vi "OverlayFGENFunctions.vi"() -> ()   [LabVIEW 2023]
doc: "This example shows how to use the Arbitrary Waveform mode to generate on two channels."
uses:
  <instrlib>/niFgen/niFgen.llb/niFgen Output Mode.ctl
  <instrlib>/niFgen/niFgen.llb/niFgen Write Waveform.vi
panel:
  in  "CH0 Waveform Information":cluster{"Waveform Type":u16, "Amplitude":dbl}={"Waveform Type"=0, "Amplitude"=1.0} {"Amplitude" min=0.0 max=1.0 format="%.2f"; "Waveform Type" items=["Sine", "Cosine", "Triangle", "Square", "Sawtooth", "Increasing Ramp", "Decreasing Ramp", "DC Value"]}
  in  "# of points":u32=256
  in  "Update":bool
  in  "Stop":bool
  in  "CH1 Gain":dbl(knob)=0.5 min=0.0 max=2.5 scale=0.0..2.5 scale format="%#.1f"
  in  "CH0 Gain":dbl(knob)=0.5 min=0.0 max=2.5 scale=0.0..2.5 scale format="%#.1f"
  in  "CH1 Waveform Information":cluster{"Waveform Type":u16, "Amplitude":dbl}={"Waveform Type"=1, "Amplitude"=1.0} {"Amplitude" min=0.0 max=1.0 format="%.2f"; "Waveform Type" items=["Sine", "Cosine", "Triangle", "Square", "Sawtooth", "Increasing Ramp", "Decreasing Ramp", "DC Value"]}
  in  "Sample Rate (S/s)":dbl=20000000.0 format="%.2p"
  in  "Sample Clock Source":string(combo)="OnboardClock"
  in  "FGEN Resource Name":refnum<k15>
  out "Waveforms":dbl[][](graph)=[[0.0, 0.024541228522912288, 0.049067674327418015, 0.07356456359966743, 0.0980171403295606, 0.1224106751992162, 0.14673047445536175, 0.17096188876030122, 0.19509032201612828, 0.2191012401568698, 0.2429801799032639, 0.26671275747489837, 0.2902846772544624, 0.31368174039889146, 0.33688985339222005, 0.3598950365349881, 0.3826834323650898, 0.40524131400498986, 0.4275550934302821, 0.4496113296546066, 0.47139673682599764, 0.49289819222978404, 0.5141027441932218, 0.5349976198870973, 0.5555702330196023, 0.5758081914178453, 0.5956993044924334, 0.6152315905806269, 0.6343932841636455, 0.6531728429537769, 0.6715589548470184, 0.689540544737067, 0.7071067811865476, 0.724247082951467, 0.7409511253549591, 0.7572088465064847, 0.773010453362737, 0.7883464276266063, 0.8032075314806449, 0.8175848131515838, 0.8314696123025452, 0.8448535652497072, 0.8577286100002721, 0.8700869911087116, 0.881921264348355, 0.8932243011955154, 0.9039892931234433, 0.9142097557035308, 0.9238795325112867, 0.9329927988347391, 0.9415440651830208, 0.9495281805930369, 0.9569403357322089, 0.9637760657954401, 0.9700312531945441, 0.9757021300385287, 0.9807852804032305, 0.9852776423889413, 0.989176509964781, 0.9924795345987101, 0.9951847266721969, 0.9972904566786903, 0.9987954562051724, 0.9996988186962044, 1.0, 0.9996988186962044, 0.9987954562051724, 0.9972904566786903, 0.9951847266721969, 0.9924795345987101, 0.989176509964781, 0.9852776423889413, 0.9807852804032305, 0.9757021300385286, 0.9700312531945441, 0.9637760657954398, 0.9569403357322089, 0.9495281805930367, 0.9415440651830208, 0.9329927988347388, 0.9238795325112867, 0.9142097557035306, 0.9039892931234433, 0.8932243011955152, 0.881921264348355, 0.8700869911087113, 0.8577286100002721, 0.844853565249707, 0.8314696123025452, 0.8175848131515836, 0.8032075314806449, 0.7883464276266061, 0.773010453362737, 0.7572088465064843, 0.7409511253549591, 0.7242470829514667, 0.7071067811865476, 0.6895405447370667, 0.6715589548470184, 0.6531728429537765, 0.6343932841636455, 0.6152315905806266, 0.5956993044924334, 0.575808191417845, 0.5555702330196023, 0.5349976198870969, 0.5141027441932218, 0.49289819222978376, 0.4713967368259977, 0.4496113296546063, 0.42755509343028214, 0.4052413140049896, 0.38268343236508984, 0.3598950365349879, 0.3368898533922201, 0.31368174039889124, 0.29028467725446244, 0.26671275747489814, 0.24298017990326395, 0.21910124015686955, 0.19509032201612833, 0.17096188876030097, 0.1467304744553618, 0.12241067519921595, 0.09801714032956065, 0.07356456359966718, 0.04906767432741806, 0.024541228522912045, 3.836381624704177e-17, -0.024541228522912528, -0.04906767432741798, -0.07356456359966766, -0.09801714032956058, -0.12241067519921643, -0.14673047445536172, -0.17096188876030144, -0.19509032201612825, -0.21910124015687, -0.24298017990326387, -0.2667127574748986, -0.29028467725446233, -0.3136817403988917, -0.33688985339222, -0.35989503653498833, -0.3826834323650897, -0.40524131400499, -0.42755509343028203, -0.44961132965460676, -0.4713967368259976, -0.4928981922297842, -0.5141027441932217, -0.5349976198870974, -0.5555702330196022, -0.5758081914178454, -0.5956993044924334, -0.6152315905806269, -0.6343932841636455, -0.6531728429537769, -0.6715589548470184, -0.689540544737067, -0.7071067811865476, -0.724247082951467, -0.7409511253549591, -0.7572088465064846, -0.773010453362737, -0.7883464276266062, -0.8032075314806449, -0.8175848131515836, -0.8314696123025452, -0.844853565249707, -0.8577286100002721, -0.8700869911087113, -0.881921264348355, -0.8932243011955152, -0.9039892931234433, -0.9142097557035306, -0.9238795325112867, -0.9329927988347388, -0.9415440651830208, -0.9495281805930366, -0.9569403357322089, -0.9637760657954397, -0.9700312531945441, -0.9757021300385283, -0.9807852804032305, -0.985277642388941, -0.989176509964781, -0.9924795345987097, -0.9951847266721969, -0.99729045667869, -0.9987954562051724, -0.999698818696204, -1.0, -0.999698818696204, -0.9987954562051724, -0.99729045667869, -0.9951847266721969, -0.9924795345987097, -0.989176509964781, -0.985277642388941, -0.9807852804032305, -0.9757021300385283, -0.9700312531945441, -0.9637760657954396, -0.9569403357322089, -0.9495281805930365, -0.9415440651830208, -0.9329927988347386, -0.9238795325112867, -0.9142097557035304, -0.9039892931234433, -0.893224301195515, -0.881921264348355, -0.8700869911087111, -0.8577286100002721, -0.8448535652497068, -0.8314696123025452, -0.8175848131515834, -0.8032075314806449, -0.7883464276266059, -0.773010453362737, -0.7572088465064842, -0.7409511253549591, -0.7242470829514666, -0.7071067811865476, -0.6895405447370666, -0.6715589548470184, -0.6531728429537764, -0.6343932841636455, -0.6152315905806265, -0.5956993044924334, -0.5758081914178449, -0.5555702330196023, -0.5349976198870968, -0.5141027441932218, -0.49289819222978365, -0.4713967368259977, -0.4496113296546062, -0.42755509343028214, -0.4052413140049895, -0.38268343236508984, -0.3598950365349878, -0.3368898533922201, -0.31368174039889113, -0.29028467725446244, -0.26671275747489803, -0.24298017990326395, -0.21910124015686946, -0.19509032201612833, -0.1709618887603009, -0.1467304744553618, -0.1224106751992159, -0.09801714032956066, -0.07356456359966715, -0.04906767432741807, -0.024541228522912028], [1.0, 0.9996988186962042, 0.9987954562051724, 0.9972904566786902, 0.9951847266721969, 0.99247953459871, 0.989176509964781, 0.9852776423889412, 0.9807852804032305, 0.9757021300385286, 0.9700312531945441, 0.9637760657954398, 0.9569403357322089, 0.9495281805930367, 0.9415440651830208, 0.9329927988347388, 0.9238795325112867, 0.9142097557035306, 0.9039892931234433, 0.8932243011955152, 0.881921264348355, 0.8700869911087113, 0.8577286100002721, 0.844853565249707, 0.8314696123025453, 0.8175848131515836, 0.803207531480645, 0.7883464276266061, 0.7730104533627371, 0.7572088465064845, 0.7409511253549592, 0.7242470829514668, 0.7071067811865477, 0.6895405447370668, 0.6715589548470186, 0.6531728429537766, 0.6343932841636456, 0.6152315905806267, 0.5956993044924335, 0.5758081914178451, 0.5555702330196024, 0.534997619887097, 0.5141027441932219, 0.49289819222978387, 0.4713967368259978, 0.44961132965460643, 0.42755509343028225, 0.4052413140049897, 0.38268343236508995, 0.359895036534988, 0.3368898533922202, 0.31368174039889135, 0.29028467725446255, 0.26671275747489825, 0.24298017990326407, 0.2191012401568697, 0.19509032201612844, 0.17096188876030113, 0.14673047445536191, 0.12241067519921611, 0.09801714032956077, 0.07356456359966734, 0.04906767432741818, 0.02454122852291222, 1.655136260252793e-16, -0.024541228522912347, -0.04906767432741785, -0.07356456359966747, -0.09801714032956044, -0.12241067519921624, -0.14673047445536158, -0.17096188876030124, -0.1950903220161281, -0.2191012401568698, -0.24298017990326373, -0.26671275747489837, -0.2902846772544622, -0.31368174039889146, -0.3368898533922199, -0.3598950365349881, -0.3826834323650896, -0.4052413140049898, -0.4275550934302819, -0.44961132965460654, -0.4713967368259975, -0.492898192229784, -0.5141027441932216, -0.5349976198870972, -0.5555702330196021, -0.5758081914178452, -0.5956993044924332, -0.6152315905806267, -0.6343932841636454, -0.6531728429537766, -0.6715589548470183, -0.6895405447370668, -0.7071067811865475, -0.7242470829514668, -0.740951125354959, -0.7572088465064843, -0.7730104533627369, -0.788346427626606, -0.8032075314806448, -0.8175848131515834, -0.8314696123025451, -0.8448535652497068, -0.857728610000272, -0.8700869911087111, -0.8819212643483549, -0.893224301195515, -0.9039892931234432, -0.9142097557035304, -0.9238795325112866, -0.9329927988347386, -0.9415440651830207, -0.9495281805930365, -0.9569403357322088, -0.9637760657954396, -0.970031253194544, -0.9757021300385283, -0.9807852804032304, -0.985277642388941, -0.989176509964781, -0.9924795345987097, -0.9951847266721969, -0.99729045667869, -0.9987954562051724, -0.999698818696204, -1.0, -0.999698818696204, -0.9987954562051724, -0.99729045667869, -0.9951847266721969, -0.9924795345987097, -0.989176509964781, -0.985277642388941, -0.9807852804032305, -0.9757021300385283, -0.9700312531945441, -0.9637760657954397, -0.9569403357322089, -0.9495281805930366, -0.9415440651830208, -0.9329927988347387, -0.9238795325112867, -0.9142097557035305, -0.9039892931234433, -0.8932243011955151, -0.881921264348355, -0.8700869911087112, -0.8577286100002721, -0.8448535652497069, -0.8314696123025453, -0.8175848131515835, -0.803207531480645, -0.7883464276266061, -0.7730104533627371, -0.7572088465064845, -0.7409511253549592, -0.7242470829514669, -0.7071067811865477, -0.6895405447370669, -0.6715589548470186, -0.6531728429537768, -0.6343932841636457, -0.6152315905806268, -0.5956993044924336, -0.5758081914178452, -0.5555702330196025, -0.5349976198870972, -0.514102744193222, -0.492898192229784, -0.4713967368259979, -0.44961132965460654, -0.42755509343028236, -0.4052413140049898, -0.38268343236509006, -0.3598950365349881, -0.33688985339222033, -0.31368174039889146, -0.29028467725446266, -0.26671275747489837, -0.24298017990326418, -0.2191012401568698, -0.19509032201612855, -0.17096188876030124, -0.14673047445536203, -0.12241067519921622, -0.09801714032956087, -0.07356456359966745, -0.04906767432741828, -0.024541228522912326, -2.6112670511134473e-16, 0.024541228522912243, 0.04906767432741776, 0.07356456359966737, 0.09801714032956035, 0.12241067519921614, 0.1467304744553615, 0.17096188876030116, 0.19509032201612803, 0.21910124015686971, 0.24298017990326365, 0.2667127574748983, 0.2902846772544621, 0.3136817403988914, 0.3368898533922198, 0.35989503653498806, 0.3826834323650895, 0.40524131400498975, 0.42755509343028186, 0.4496113296546065, 0.4713967368259974, 0.4928981922297839, 0.5141027441932216, 0.534997619887097, 0.5555702330196021, 0.5758081914178451, 0.5956993044924332, 0.6152315905806267, 0.6343932841636454, 0.6531728429537766, 0.6715589548470183, 0.6895405447370668, 0.7071067811865475, 0.7242470829514668, 0.740951125354959, 0.7572088465064845, 0.7730104533627369, 0.7883464276266061, 0.8032075314806448, 0.8175848131515836, 0.8314696123025451, 0.844853565249707, 0.857728610000272, 0.8700869911087113, 0.8819212643483549, 0.8932243011955152, 0.9039892931234432, 0.9142097557035306, 0.9238795325112866, 0.9329927988347388, 0.9415440651830207, 0.9495281805930367, 0.9569403357322088, 0.9637760657954398, 0.970031253194544, 0.9757021300385286, 0.9807852804032304, 0.9852776423889412, 0.989176509964781, 0.99247953459871, 0.9951847266721969, 0.9972904566786902, 0.9987954562051724, 0.9996988186962042]]
  # "Overview: Demonstrates the Arbitrary Waveform output mode to generate waveforms on two channel devices.\nSoftware Requirements: NI-FGEN\nHardware Requirements:  NI PXIe-5413, NI PXIe-5423, NI PXIe-5433, NI PXIe-5450, NI PXIe-5451 \nInstructions:\n1. Select the FGEN Resource Name as configured in the Measurement & Automation Explorer.\n2. Select the Sample Clock Source that will be used.\n3. Specify the Sample Rate (S/s) that will be used.\n4. Specify the waveform that will be generated on CH0 with CH0 Waveform Information.\n5. Specify the waveform that will be generated on CH1 with CH1 Waveform Information.\n6. Specify the # of points that both waveforms will have.\n7. Specify the gain on CH0 with CH0 Gain and the gain on CH1 with CH1 Gain that will be used.\n8. Run the VI.\n9. You can change the CH0 Gain or CH1 Gain values on-the-fly. If you want to update any other parameter, click Update to abort the current generation task and to restart the generation with the new configuration of the NI Function Generator.\n10. Click Stop to stop the VI."
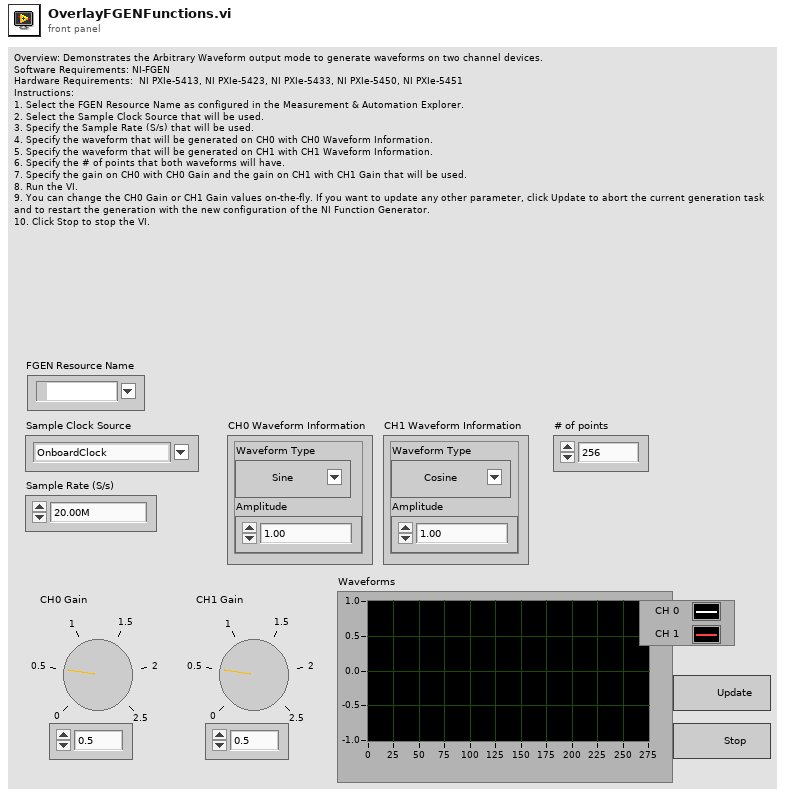
[diagram p1: front panel]
types:
  T1 = typedef "niFgen Output Mode.ctl" = u32
  T2 = cluster{"Waveform Type":u16, dbl, "# of points":u32}
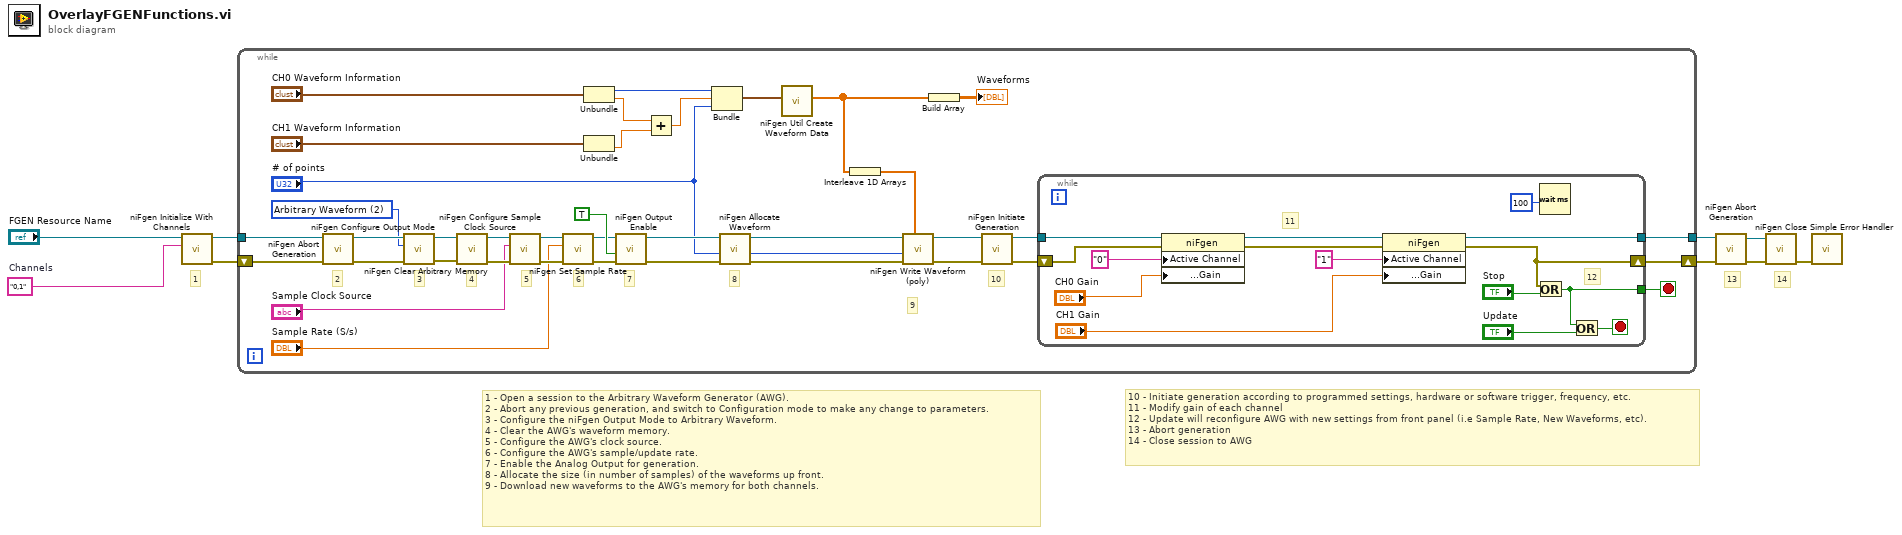
[diagram p0: block diagram]
diagram:
  w3 = "0,1"  # Channels
  # "14"
  # "13"
  # "1"
  # "1 - Open a session to the Arbitrary Waveform Generator (AWG).\n2 - Abort any previous generation, and switch to Configuration mode to make any change to parameters.\n3 - Configure the niFgen Output Mode to Arbitrary Waveform.\n4 - Clear the AWG's waveform memory.\n5 - Configure the AWG's clock source.\n6 - Configure the AWG's sample/update rate.\n7 - Enable the Analog Output for generation.\n8 - Allocate the size (in number of samples) of the waveforms up front.\n9 - Download new waveforms to the AWG's memory for both channels."
  # "10 - Initiate generation according to programmed settings, hardware or software trigger, frequency, etc.\n11 - Modify gain of each channel \n12 - Update will reconfigure AWG with new settings from front panel (i.e Sample Rate, New Waveforms, etc).\n13 - Abort generation\n14 - Close session to AWG"
  n1 = call <instrlib>:"niFgen Initialize With Channels.vi"("Channel Name"=w3, "Resource Name"="FGEN Resource Name") -> ("error out"=w2:errorcluster, "Instrument Handle Out"=w1:refnum<k15>)  [unwired: 8 in]
  n2 = while {
    tunnel: [w48] -> w9
    tunnel: w1 -> [w47]
    shift-right: [w16] -> w5
    shift-left: w2 -> [w38]
    stop <- w17 stop-if-true
    w44 = T1 2 items=["Standard Function", "Frequency List", "Arbitrary Waveform", "Arbitrary Sequence", "Script"] ("Output Mode")
    # "10"
    # "9"
    # "7"
    # "8"
    # "6"
    # "5"
    # "4"
    # "3"
    # "2"
    n3 = call <instrlib>:"niFgen Abort Generation.vi"("error in (no error)"=w38, "Instrument Handle"=w47) -> ("error out"=w46:errorcluster, "Instrument Handle Out"=w45:refnum<k15>)  [unwired: 8 in]
    n4 = call <instrlib>:"niFgen Configure Output Mode.vi"("error in (no error)"=w46, "Output Mode (default: 0=Standard Function)"=w44, "Instrument Handle"=w45) -> ("error out"=w42:errorcluster, "Instrument Handle Out"=w43:refnum<k15>)  [unwired: 6 in]
    n5 = call <instrlib>:"niFgen Clear Arbitrary Memory.vi"("error in (no error)"=w42, "Instrument Handle"=w43) -> ("error out"=w30:errorcluster, "Instrument Handle Out"=w31:refnum<k15>)  [unwired: 8 in]
    n6 = call <instrlib>:"niFgen Configure Sample Clock Source.vi"("error in (no error)"=w30, "Source (Onboard Clock)"="Sample Clock Source", "Instrument Handle"=w31) -> ("error out"=w40:errorcluster, "Instrument Handle Out"=w41:refnum<k15>)  [unwired: 7 in]
    n7 = call <instrlib>:"niFgen Set Sample Rate.vi"("error in (no error)"=w40, "Sample Rate (Samp/s)"="Sample Rate (S/s)", "Instrument Handle"=w41) -> ("error out"=w27:errorcluster, "Instrument Handle Out"=w28:refnum<k15>)  [unwired: 7 in]
    n8 = Unbundle("CH0 Waveform Information") -> ("Waveform Type"=w10:u16, "Amplitude"=w12:dbl)
    n9 = Unbundle("CH1 Waveform Information") -> ("Amplitude"=w13:dbl)  [unwired: 1 out]
    n10 = call <instrlib>:"niFgen Output Enable.vi"("error in (no error)"=w27, "Output Enable (default: True)"=TRUE ("output enable"), "Instrument Handle"=w28) -> ("error out"=w35:errorcluster, "Instrument Handle Out"=w34:refnum<k15>)  [unwired: 7 in]
    n11 = Add(x=w12, y=w13) -> (x+y=w11:dbl)
    n12 = Bundle("Waveform Type"=w10, w11, "# of points"="# of points") -> (w29:T2)  [unwired: 1 in]
    n13 = call <instrlib>:"niFgen Allocate Waveform.vi"("error in (no error)"=w35, "Waveform Size"="# of points", "Instrument Handle"=w34) -> ("error out"=w33:errorcluster, "Waveform Handle Out"=w36:i32, "Instrument Handle Out"=w32:refnum<k15>)  [unwired: 6 in]
    n14 = call <instrlib>:"niFgen Util Create Waveform Data.vi"("Waveform"=w29) -> ("Waveform Data"=w15:dbl[])  [unwired: 10 in]
    n15 = Interleave 1D Arrays(w15) -> (w14:dbl[])
    n16 = call-poly <instrlib>:"niFgen Write Waveform (poly).vi"("Waveform Data"=w14, "error in (no error)"=w33, "Waveform Handle"=w36, "Instrument Handle"=w32) -> ("error out"=w25:errorcluster, "Instrument Handle Out"=w26:refnum<k15>)  [unwired: 5 in, 1 out]
    n17 = Build Array(w15) -> (→"Waveforms":dbl[][])
    n18 = call <instrlib>:"niFgen Initiate Generation.vi"("error in (no error)"=w25, "Instrument Handle"=w26) -> ("error out"=w23:errorcluster, "Instrument Handle Out"=w24:refnum<k15>)  [unwired: 8 in]
    n19 = while {
      tunnel: [w55] -> w48
      tunnel: w24 -> [w61]
      tunnel: [w49] -> w17
      shift-right: [w54] -> w16
      shift-left: w23 -> [w60]
      stop <- w62 stop-if-true
      # "11"
      # "12"
      n20 = property class="niFgen"(reference=w61, error in=w60, "Active Channel"="0", "Arbitrary Waveform:Gain"="CH0 Gain") -> (reference out=w58:refnum<k15>, error out=w57:errorcluster)
      n21 = property class="niFgen"(reference=w58, error in=w57, "Active Channel"="1", "Arbitrary Waveform:Gain"="CH1 Gain") -> (reference out=w55:refnum<k15>, error out=w54:errorcluster)
      n22 = Or(x=w54, y="Stop") -> (x .or. y?=w49:bool)
      n23 = Wait (ms)(milliseconds to wait=u32 100 ("millisecond multiple")) -> ()  [unwired: 1 out]
      n24 = Or(x=w49, y="Update") -> (x .or. y?=w62:bool)
    }
  }
  n25 = call <instrlib>:"niFgen Abort Generation.vi"("error in (no error)"=w5, "Instrument Handle"=w9) -> ("error out"=w8:errorcluster, "Instrument Handle Out"=w7:refnum<k15>)  [unwired: 8 in]
  n26 = call <instrlib>:"niFgen Close.vi"("error in (no error)"=w8, "Instrument Handle"=w7) -> ("error out"=w6:errorcluster)  [unwired: 9 in]
  n27 = call <vilib>:"Simple Error Handler.vi"("error in (no error)"=w6) -> ()  [unwired: 4 in, 5 out]
